vi "MeasurementItems_SetChannels.vi"(8 "error in (no error)":errorcluster, 10 "Channel Name List":string[](array[string]), 11 "OXY_SCPI Reseource In":refnum<visa-resource-name>) -> (0 "error out":errorcluster, 1 "communication_data":T1, 3 "OXY_SCPI Reseource Out":refnum<visa-resource-name>)   [LabVIEW 2018, in "OXYGEN.lvlib"]
doc: "Set numeric data output items."
uses:
  OXYGEN.lvlib
  TypeDefs/Cluster_RawCommData.ctl
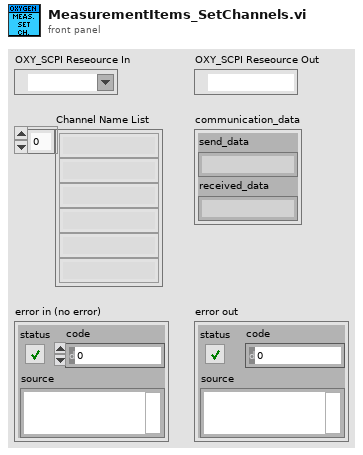
[diagram p1: front panel]
types:
  T1 = typedef "OXYGEN.lvlib/Cluster_RawCommData.ctl" = cluster{"send_data":string, "received_data":string}
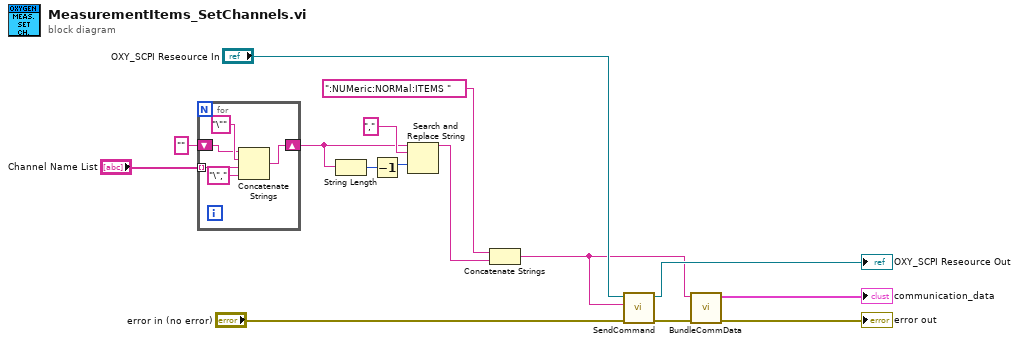
[diagram p0: block diagram]
diagram:
  n1 = for {
    tunnel: "Channel Name List" -> [w20] mode=indexing
    shift-right: [w17] -> w11
    shift-left: "" -> [w16]
    n2 = Concatenate Strings(w16, "\"" ("string"), w20, "\"," ("string")) -> (w17:string)
  }
  n3 = String Length(string=w11) -> (length=w10:i32)
  n4 = Decrement(x=w10) -> (x-1=w13:i32)
  n5 = Search and Replace String(input string=w11, search string=",", offset=w13) -> (result string=w1:string)  [unwired: 5 in, 3 out]
  n6 = Concatenate Strings(":NUMeric:NORMal:ITEMS " ("string"), w1) -> (w3:string)
  n7 = call "SendCommand.vi"("error in (no error)"="error in (no error)", "String to Send"=w3, "OXY_SCPI Reseource In"="OXY_SCPI Reseource In") -> ("error out"=w4:errorcluster, "OXY_SCPI Reseource Out"=→"OXY_SCPI Reseource Out":refnum<visa-resource-name>)  [unwired: 7 in]
  n8 = call "BundleCommData.vi"("error in (no error)"=w4, "send_data"=w3) -> ("error out"=→"error out":errorcluster, "communication_data"=→"communication_data":T1)  [unwired: 8 in]
